vi "minusOne.vi"(8 "error in (no error)":errorcluster, 11 "NPad2 in":refnum<class "NPad2.lvclass">) -> (0 "error out":errorcluster, 3 "NPad2 out":refnum<class "NPad2.lvclass">)   [LabVIEW 2020, in "NPad2.lvlib" / "NPad2.lvclass"]
uses:
  NPad2.lvclass
  NPad2.lvclass/NPad2.ctl
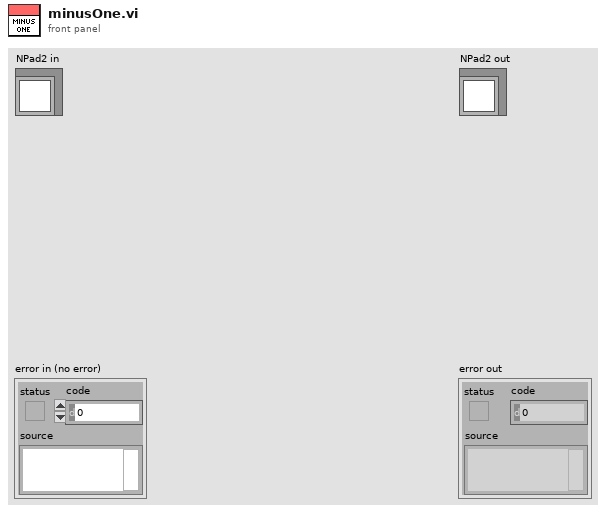
[diagram p1: front panel]
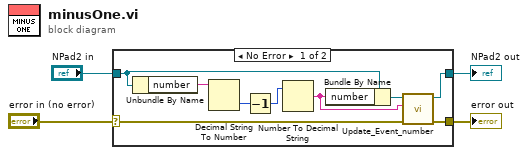
[diagram p0: block diagram]
diagram:
  n1 = case shown="No Error" "error in (no error)" {
    selector: "error in (no error)" -> [w6 w15]
    tunnel: [w5 w15] -> w3
    tunnel: [w8 w14] -> w1
    tunnel: "NPad2 in" -> [w10 w14]
    frame No Error {
      n2 = Unbundle By Name(w10) -> ("number"=w13:string)
      n3 = Decimal String To Number(string=w13) -> (number=w12:i32)  [unwired: 2 in, 1 out]
      n4 = Decrement(x=w12) -> (x-1=w11:i32)
      n5 = Number To Decimal String(number=w11) -> (decimal integer string=w7:string)  [unwired: 1 in]
      n6 = Bundle By Name(cluster=w10, "number"=w7) -> (w9:refnum<class "NPad2.lvclass">)
      n7 = call "Update_Event_number.vi"("error in (no error)"=w6, "number"=w7, "NPad2 in"=w9) -> ("error out"=w5:errorcluster, "NPad2 out"=w8:refnum<class "NPad2.lvclass">)  [unwired: 7 in]
    }
    frame Error {
    }
  }
  "error out" <- w3
  "NPad2 out" <- w1
